vi "init.vi"(3 "Container State":T5, 4 "Previous State":variant, 5 "Previous Version":T4) -> (2 "Current State":T1={"control refs"={"z offset"=refnum, "laser intensity"=refnum, "XY graph"=refnum}, "error"={"status"=FALSE, "code"=0, "source"=""}, "free-run?"=TRUE, "settings"={"fix points"=[], "A"=0.0, "lambda"=0.0, "C"=0.0}, "range (um)"=0, "interpolate?"=FALSE})   [LabVIEW 2010, in "XIntensityCompensation.xctl"]
uses:
  XIntensityCompensation.xctl
  state.ctl
  control_refs.ctl
  settings_cluster.ctl
  <vilib>/_xctls/Container State.ctl
  <vilib>/_xctls/Version.ctl
  <vilib>/_xctls/XControlSupport.lvlib
panel:
  in  "Default Indicator State":T1={"control refs"={"z offset"=refnum, "laser intensity"=refnum, "XY graph"=refnum}, "error"={"status"=FALSE, "code"=0, "source"=""}, "free-run?"=TRUE, "settings"={"fix points"=[], "A"=0.0, "lambda"=0.0, "C"=0.0}, "range (um)"=0, "interpolate?"=FALSE}
  in  "Default Control State":T1={"control refs"={"z offset"=refnum, "laser intensity"=refnum, "XY graph"=refnum}, "error"={"status"=FALSE, "code"=0, "source"=""}, "free-run?"=TRUE, "settings"={"fix points"=[], "A"=0.0, "lambda"=0.0, "C"=0.0}, "range (um)"=0, "interpolate?"=FALSE}
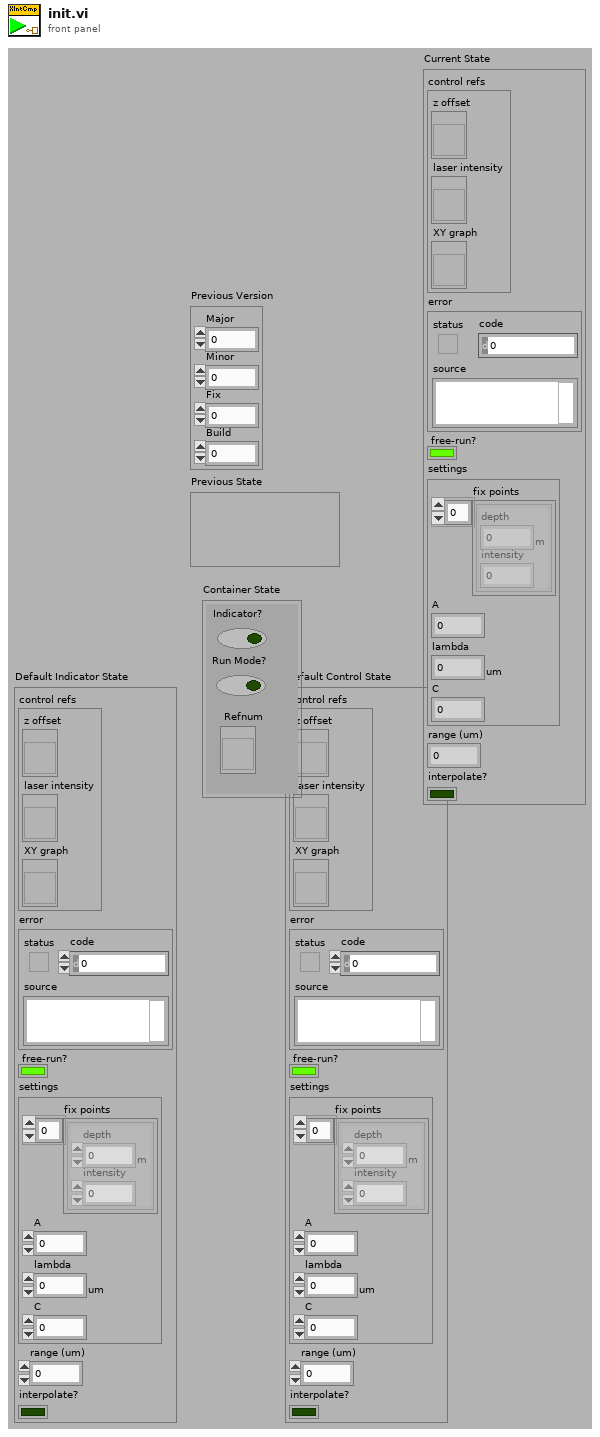
[diagram p1: front panel]
types:
  T1 = typedef "XIntensityCompensation.xctl/state.ctl" = cluster{"control refs":T2, "error":errorcluster, "free-run?":bool, "settings":T3, "range (um)":i32, "interpolate?":bool}
  T2 = typedef "XIntensityCompensation.xctl/control_refs.ctl" = cluster{"z offset":refnum<vi>, "laser intensity":refnum<vi>, "XY graph":refnum<vi>}
  T3 = typedef "XIntensityCompensation.xctl/settings_cluster.ctl" = cluster{"fix points":cluster{"depth":dbl[unit], "intensity":dbl}[], "A":dbl, "lambda":dbl[unit], "C":dbl}
  T4 = typedef "XControlSupport.lvlib/Version.ctl" = cluster{"Major":u16, "Minor":u16, "Fix":u16, "Build":u16}
  T5 = typedef "XControlSupport.lvlib/Container State.ctl" = cluster{"Indicator?":bool, "Run Mode?":bool, " Refnum":refnum<vi>}
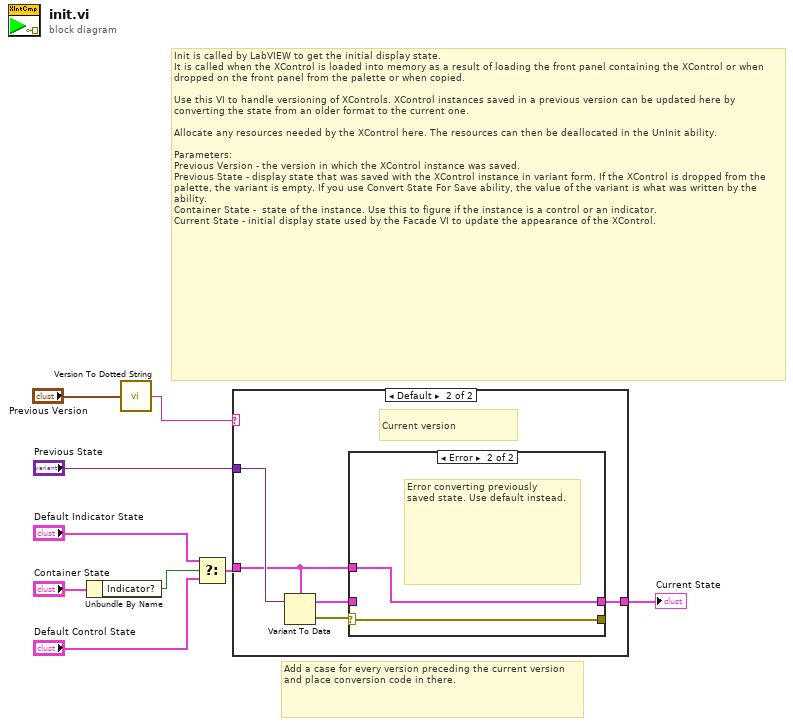
[diagram p0: block diagram]
diagram:
  # "Add a case for every version preceding the current version and place conversion code in there."
  # "Init is called by LabVIEW to get the initial display state.\nIt is called when the XControl is loaded into memory as a result of loading the front panel containing the XControl or when dropped on the front panel from the palette or when copied.\n\nUse this VI to handle versioning of XControls. XControl instances saved in a previous version can be updated here by converting the state from an older format to the current one.\n\nAllocate any resources needed by the XControl here. The resources can then be deallocated in the UnInit ability.\n\nParameters:\nPrevious Version - the version in which the XControl instance was saved.\nPrevious State - display state that was saved with the XControl instance in variant form. If the XControl is dropped from the palette, the variant is empty. If you use Convert State For Save ability, the value of the variant is what was written by the ability. \nContainer State -  state of the instance. Use this to figure if the instance is a control or an indicator.\nCurrent State - initial display state used by the Facade VI to update the appearance of the XControl."
  n1 = Unbundle By Name("Container State") -> ("Indicator?"=w4:bool)
  n2 = call <vilib>:"Version To Dotted String.vi"("Version"="Previous Version") -> ("String Version"=w1:string)
  n3 = Select(t="Default Indicator State", s=w4, f="Default Control State") -> (s? t:f=w3:T1)
  n4 = case shown="Default" w1 {
    tunnel: "Previous State" -> [_ w15]
    tunnel: [w10 w11] -> w8
    tunnel: w3 -> [w10 w12]
    frame "0.0.0.0" {
      # "Just created, use default state"
    }
    frame Default {
      # "Current version"
      n5 = Variant To Data(Variant=w15, type=w12) -> (error out=w14:errorcluster, data=w13:T1)  [unwired: 1 in]
      n6 = case shown="Error" w14 {
        selector: w14 -> [w17 w18]
        tunnel: w13 -> [w16 _]
        tunnel: [w16 w19] -> w11
        tunnel: w12 -> [_ w19]
        tunnel: [w17 w18] -> _
        frame No Error {
        }
        frame Error {
          # "Error converting previously \nsaved state. Use default instead."
        }
      }
    }
  }
  "Current State" <- w8
